vi "Test Maui 2.0.vi"(8 "error in":errorcluster) -> (0 "error out":errorcluster)   [LabVIEW 2020]
uses:
  <vilib>/addons/_JKI Toolkits/Caraya/classes/Test/Test.lvclass
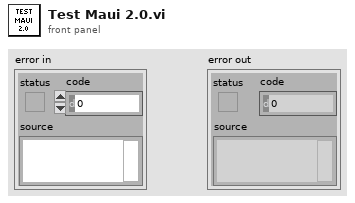
[diagram p1: front panel]
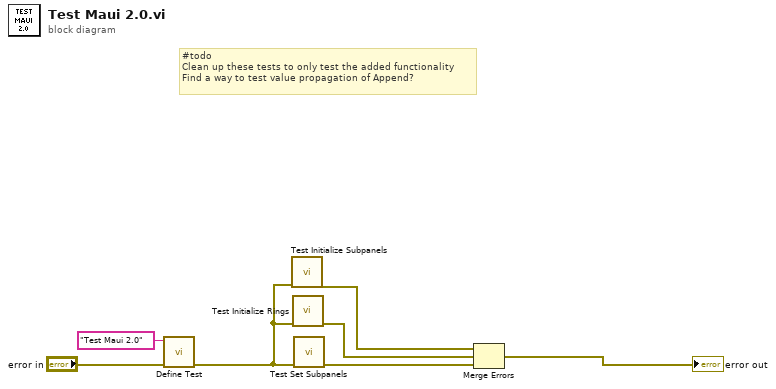
[diagram p0: block diagram]
diagram:
  # "#todo\nClean up these tests to only test the added functionality\nFind a way to test value propagation of Append?"
  n1 = call <vilib>:"Define Test.vi"("error in (no error)"="error in", "Label (VI Title)"="Test Maui 2.0") -> ("error out"=w2:errorcluster)  [unwired: 9 in]
  n2 = call "Test Initialize Subpanels.vi"("error in"=w2) -> ("error out"=w1:errorcluster)  [unwired: 10 in]
  n3 = call "Test Initialize Rings.vi"("error in"=w2) -> ("error out"=w3:errorcluster)  [unwired: 10 in]
  n4 = call "Test Set Subpanels.vi"("error in"=w2) -> ("error out"=w4:errorcluster)  [unwired: 10 in]
  n5 = Merge Errors(w1, w3, w4) -> (→"error out":errorcluster)
